vi "Initialize.vi"(8 "error in":errorcluster) -> (0 "error out":errorcluster, 3 "ChanMngOOB_Rx out":refnum<class "ChanMngOOB_Rx.lvclass">)   [LabVIEW 2021, in "ChanMngOOB_Rx.lvclass"]
uses:
  ChanMngOOB_Rx.lvclass
  <vilib>/CIF Foundation/CIF Out of Band Commands/CIFOutOfBand.lvclass
  Typedef/Template Payload.ctl
  C:/Program Files/National Instruments/LabVIEW 2021/vi.lib/CIF Foundation/CIF Out of Band Commands/CIFOutOfBand.lvclass
  Typedef/Channel Connection Data.ctl
  Typedef/Channel Fault Data.ctl
  <vilib>/CIF Foundation/CIF Channels Core/ChannelCommon/typedef/New FIFO Instance Configuration.ctl
  <vilib>/CIF Foundation/CIF Channels Core/ChannelCommon/ChannelCommon.lvlib
  Typedef/FIFO Publisher.ctl
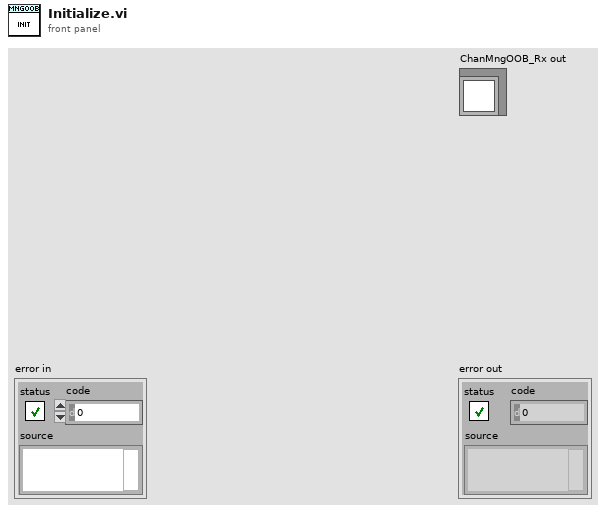
[diagram p1: front panel]
types:
  T1 = typedef "ChanMngOOB_Rx.lvclass/Channel Fault Data.ctl" = cluster{"Channel Name":string, "Force Data":u8[], "Force Active":bool}
  T2 = typedef "ChanMngOOB_Rx.lvclass/Channel Connection Data.ctl" = cluster{"Publisher Name":string, "Subscriber Name":string, "Connection Data":u8[]}
  T3 = typedef "ChanMngOOB_Rx.lvclass/Template Payload.ctl" = cluster{"Connections":T2[], "Forces":T1[], "FIFO Pub":T4}
  T4 = typedef "ChanMngOOB_Rx.lvclass/FIFO Publisher.ctl" = cluster{"Publisher Name":string, "New FIFO Instance Config":T5}
  T5 = typedef "ChannelCommon.lvlib/New FIFO Instance Configuration.ctl" = cluster{"Primary":bool, "Backpressure":bool, "Message/FIFO Override":u32}
  T6 = typedef "ChanMngOOB_Rx.lvclass/Command Setting Control.ctl" = cluster{"Enum":T7, "U8":u8, " Payload":bool}
  T7 = typedef "ChanMngOOB_Rx.lvclass/OOB ChnMng Commands.ctl" = enum8{"Connect Channel", "Force Channel", "Add FIFO Pub", "Remove FIFO Pub"}
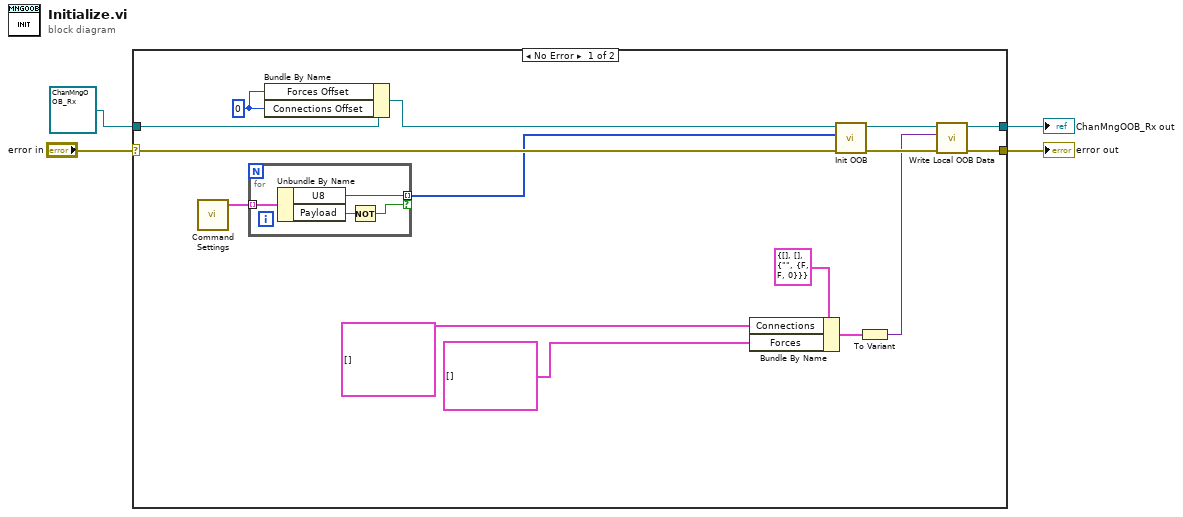
[diagram p0: block diagram]
diagram:
  n1 = case shown="No Error" "error in" {
    selector: "error in" -> [w19 w25]
    tunnel: [w13 w25] -> w3
    tunnel: [w14 w24] -> w2
    tunnel: refnum<class "ChanMngOOB_Rx.lvclass"> refnum ("CifLvTemplateOutOfBand in") -> [w9 w24]
    frame No Error {
      w6 = 0 ("Connections Offset")
      n2 = call "Command Settings.vi"() -> ("Command Settings"=w18:T6[])  [unwired: 5 in]
      n3 = for {
        tunnel: w18 -> [w23] mode=indexing
        tunnel: [w22] -> w17 mode=indexing if=w20
        n4 = Unbundle By Name(w23) -> ("U8"=w22:u8, "Payload"=w21:bool)
        n5 = Not(x=w21) -> (.not. x?=w20:bool)
      }
      n6 = Bundle By Name(cluster=w9, "Forces Offset"=w6, "Connections Offset"=w6) -> (w8:refnum<class "ChanMngOOB_Rx.lvclass">)
      n7 = Bundle By Name(cluster=T3 {"Connections"=[], "Forces"=[], "FIFO Pub"={"Publisher Name"="", "New FIFO Instance Config"={"Primary"=FALSE, "Backpressure"=FALSE, "Message/FIFO Override"=0}}} ("Template Payload"), "Connections"=T2[] [], "Forces"=T1[] [] ("Faults")) -> (w11:T3)
      n8 = call <vilib>:"Init OOB.vi"("error in (no error)"=w19, "Cases to Skip Payload"=w17, "OOB in"=w8) -> ("error out"=w16:errorcluster, "OOB out"=w15:refnum<class "ChanMngOOB_Rx.lvclass">)  [unwired: 7 in]
      n9 = To Variant(anything=w11) -> (Variant=w10:variant)
      n10 = call <vilib>:"Write Local OOB Data.vi"("error in"=w16, "Local OOB Data"=w10, "OOB in"=w15) -> ("error out"=w13:errorcluster, "OOB out"=w14:refnum<class "ChanMngOOB_Rx.lvclass">)  [unwired: 7 in]
    }
    frame Error {
    }
  }
  "error out" <- w3
  "ChanMngOOB_Rx out" <- w2
